vi "FL Function Plot.vi"(7 "Function":T1 items=["Triangle", "Trapezoid", "Singleton", "Sigmoid", "Gaussian", "User-Defined"], 10 "Points":dbl[](array[numeric])) -> (2 "Function Graph":cluster{dbl, dbl}[](graph))   [LabVIEW 2013, in "NI_Fuzzy_Logic_API.lvlib"]
uses:
  <vilib>/addons/Fuzzy Logic/NI_Fuzzy_Logic_API.lvlib
  <vilib>/addons/Fuzzy Logic/TypeDefs/FL Membership Function Shape.ctl
  <vilib>/gmath/NI_Gmath.lvlib
panel:
  # "This VI creates a visual plot data for a function defined by 1, 3 or 4 points."
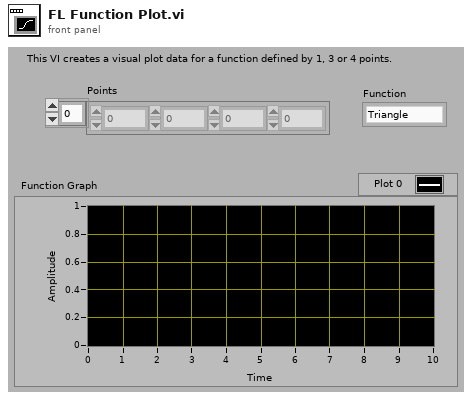
[diagram p1: front panel]
types:
  T1 = typedef "NI_Fuzzy_Logic_API.lvlib/FL Membership Function Shape.ctl" = u16
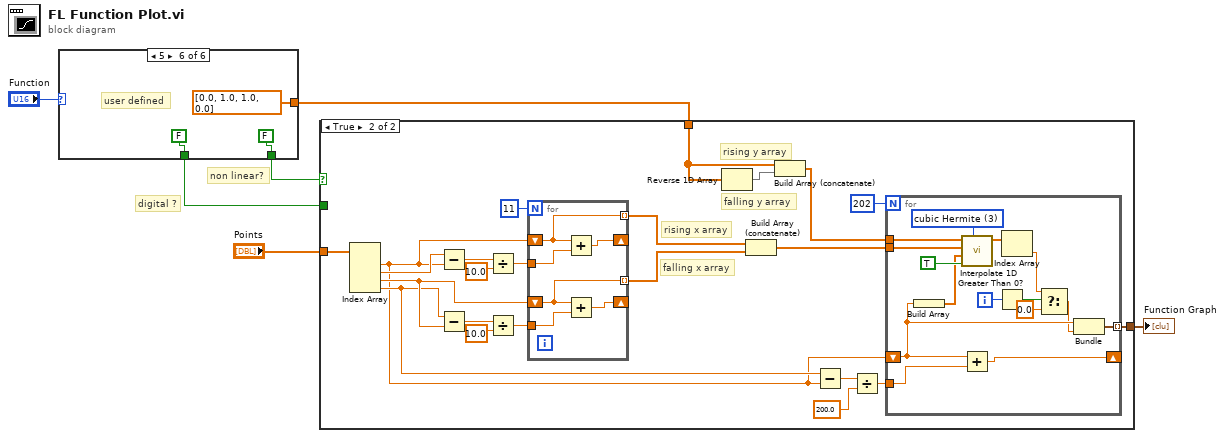
[diagram p0: block diagram]
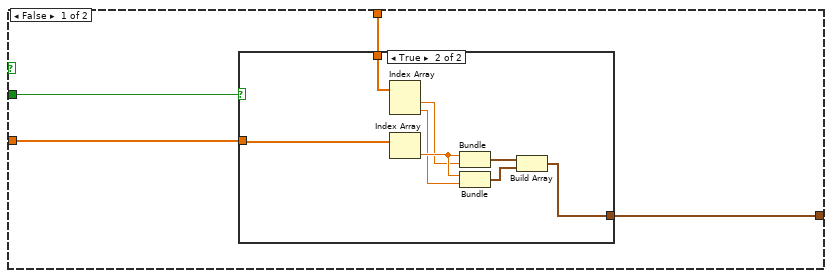
[diagram p2: hidden frame]
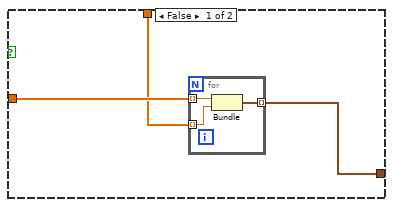
[diagram p3: hidden frame]
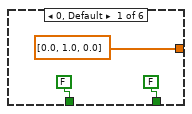
[diagram p4: hidden frame]
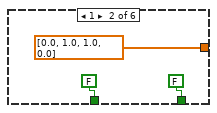
[diagram p5: hidden frame]
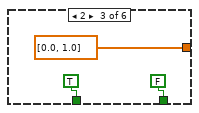
[diagram p6: hidden frame]
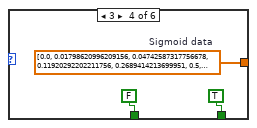
[diagram p7: hidden frame]
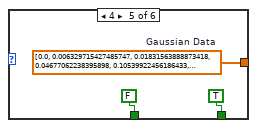
[diagram p8: hidden frame]
diagram:
  # "digital ?"
  # "non linear?"
  n1 = case shown="5" "Function" {
    tunnel: [dbl[] [0.0, 1.0, 0.0] ("Points") dbl[] [0.0, 1.0, 1.0, 0.0] ("Points") dbl[] [0.0, 1.0] ("Gaussian Data") w18 w21 dbl[] [0.0, 1.0, 1.0, 0.0] ("Gaussian Data")] -> w4
    tunnel: [FALSE FALSE FALSE TRUE TRUE FALSE] -> w2
    tunnel: [FALSE FALSE TRUE FALSE FALSE FALSE] -> w1
    frame 0, Default {
    }
    frame 1 {
    }
    frame 2 {
    }
    frame 3 {
      w18 = dbl[] [0.0, 0.01798620996209156, 0.04742587317756678, 0.11920292202211756, 0.2689414213699951, 0.5, 0.7310585786300049, 0.8807970779778824, 0.9525741268224333, 0.9820137900379085, 1.0]  # Sigmoid data
    }
    frame 4 {
      w21 = dbl[] [0.0, 0.006329715427485747, 0.01831563888873418, 0.04677062238395898, 0.10539922456186433, 0.2096113871510978, 0.36787944117144233, 0.569782824730923, 0.7788007830714049, 0.9394130628134758, 1.0]  # Gaussian Data
    }
    frame 5 {
      # "user defined"
    }
  }
  n2 = case shown="True" w2 {
    tunnel: "Points" -> [w28 w65]
    tunnel: [w26 w43] -> w5
    tunnel: w4 -> [w27 w44]
    tunnel: w1 -> [w25 _]
    frame False {
      n3 = case shown="True" w25 {
        tunnel: w28 -> [w31 w39]
        tunnel: w27 -> [w30 w37]
        tunnel: [w29 w38] -> w26
        frame False {
          n4 = for {
            tunnel: w31 -> [w34] mode=indexing
            tunnel: w30 -> [w33] mode=indexing
            tunnel: [w32] -> w29 mode=indexing
            n5 = Bundle("Xmin"=w34, "Numeric"=w33) -> (w32:cluster{"Xmin":dbl, "Numeric":dbl})  [unwired: 1 out]
          }
        }
        frame True {
          n6 = Index Array(array=w37) -> (element #1=w36:dbl, element #2=w35:dbl)  [unwired: 2 in]
          n7 = Index Array(array=w39) -> (element=w42:dbl)  [unwired: 1 in]
          n8 = Bundle("Xmin"=w42, "Numeric"=w36) -> (w41:cluster{"Xmin":dbl, "Numeric":dbl})  [unwired: 1 out]
          n9 = Bundle("Xmin"=w42, "Numeric"=w35) -> (w40:cluster{"Xmin":dbl, "Numeric":dbl})  [unwired: 1 out]
          n10 = Build Array(w41, w40) -> (w38:cluster{"Xmin":dbl, "Numeric":dbl}[])
        }
      }
    }
    frame True {
      # "falling y array"
      # "rising y array"
      # "falling x array"
      # "rising x array"
      n11 = Index Array(array=w65) -> (element #1=w48:dbl, element #2=w64:dbl, element #3=w57:dbl, element #4=w52:dbl)  [unwired: 4 in]
      n12 = Subtract(x=w64, y=w48) -> (x-y=w63:dbl)
      n13 = Subtract(x=w52, y=w57) -> (x-y=w58:dbl)
      n14 = Divide(x=w63, y=10.0) -> (x/y=w61:dbl)
      n15 = Divide(x=w58, y=10.0) -> (x/y=w56:dbl)
      n16 = for {
        N: 11 -> [_]
        tunnel: w61 -> [w86]
        shift-right: [w85] -> _
        shift-left: w48 -> [w84]
        tunnel: [w84] -> w54 mode=indexing
        tunnel: w56 -> [w83]
        shift-right: [w82] -> _
        shift-left: w57 -> [w81]
        tunnel: [w81] -> w55 mode=indexing
        n17 = Add(x=w84, y=w86) -> (x+y=w85:dbl)
        n18 = Add(x=w81, y=w83) -> (x+y=w82:dbl)
      }
      n19 = Reverse 1D Array(array=w44) -> (reversed array=w53:dbl[])
      n20 = Build Array (concatenate)(w54, w55) -> (w46:dbl[])
      n21 = Build Array (concatenate)(w44, w53) -> (w47:dbl[])
      n22 = Subtract(x=w52, y=w48) -> (x-y=w51:dbl)
      n23 = Divide(x=w51, y=200.0) -> (x/y=w49:dbl)
      n24 = for {
        N: 202 -> [_]
        tunnel: w46 -> [w77]
        tunnel: w47 -> [w76]
        tunnel: w49 -> [w75]
        shift-right: [w74] -> _
        shift-left: w48 -> [w69]
        tunnel: [w72] -> w43 mode=indexing
        i -> [w71]
        w73 = 3 items=["nearest", "linear", "spline", "cubic Hermite", "Lagrange"] ("method")
        n25 = Build Array(w69) -> (w79:dbl[])
        n26 = call <vilib>:"Interpolate 1D.vi"("method"=w73, "X is monotonic"=TRUE, "xi"=w79, "X"=w77, "Y"=w76) -> ("yi"=w78:dbl[])  [unwired: 1 in, 5 out]
        n27 = Add(x=w69, y=w75) -> (x+y=w74:dbl)
        n28 = Greater Than 0?(x=w71) -> (x > 0?=w70:bool)
        n29 = Index Array(array=w78) -> (element=w67:dbl)  [unwired: 1 in]
        n30 = Select(t=w67, s=w70, f=0.0 ("t")) -> (s? t:f=w68:dbl)
        n31 = Bundle("Xmin"=w69, "t"=w68) -> (w72:cluster{"Xmin":dbl, "t":dbl})  [unwired: 1 out]
      }
    }
  }
  "Function Graph" <- w5
